vi "save_metadata.vi"(10 "input cluster":T1, 11 "Pasta Destino":path=path "D:/labview_ieav/acquisition") -> ()   [LabVIEW 2020]
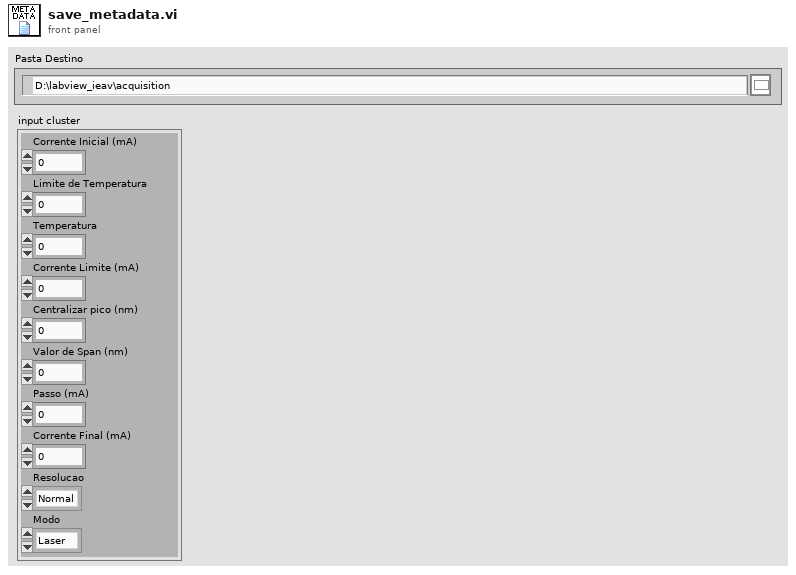
[diagram p1: front panel]
types:
  T1 = cluster{"Corrente Inicial (mA)":dbl, "Limite de Temperatura":dbl, "Temperatura":dbl, "Corrente Limite (mA)":i32, "Centralizar pico (nm)":dbl, "Valor de Span (nm)":dbl, "Passo (mA)":dbl, "Corrente Final (mA)":dbl, "Resolucao":enum16{"Normal", "High"}, "Modo":enum16{"Laser", "Led"}}
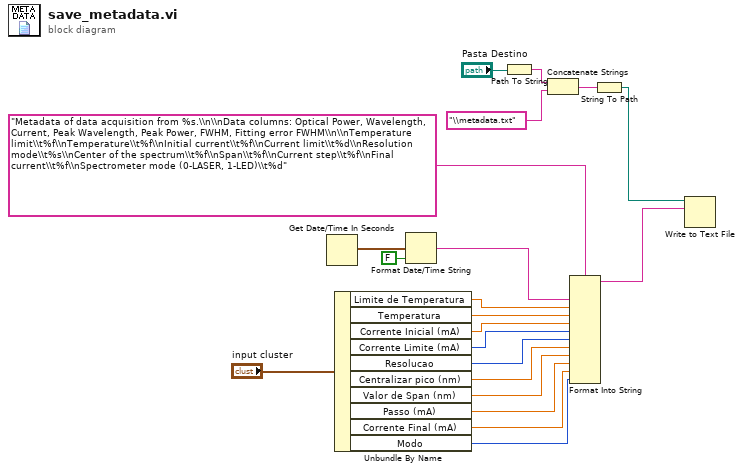
[diagram p0: block diagram]
diagram:
  n1 = Get Date/Time In Seconds() -> (seconds since 1Jan1904=w20:timestamp)
  n2 = Unbundle By Name("input cluster") -> ("Limite de Temperatura"=w18:dbl, "Temperatura"=w17:dbl, "Corrente Inicial (mA)"=w16:dbl, "Corrente Limite (mA)"=w15:i32, "Resolucao"=w14:enum16{"Normal", "High"}, "Centralizar pico (nm)"=w13:dbl, "Valor de Span (nm)"=w12:dbl, "Passo (mA)"=w11:dbl, "Corrente Final (mA)"=w10:dbl, "Modo"=w2:enum16{"Laser", "Led"})
  n3 = Format Date/Time String(seconds (now)=w20, UTC format=FALSE) -> (date/time string=w19:string)  [unwired: 1 in]
  n4 = Path To String(path="Pasta Destino") -> (string=w7:string)
  n5 = Concatenate Strings(w7, "\\metadata.txt") -> (w5:string)
  n6 = Format Into String(format string="Metadata of data acquisition from %s.\\n\\nData columns: Optical Power, Wavelength, Current, Peak Wavelength, Peak Power, FWHM, Fitting error FWHM\\n\\nTemperature limit\\t%f\\nTemperature\\t%f\\nInitial current\\t%f\\nCurrent limit\\t%d\\nResolution mode\\t%s\\nCenter of the spectrum\\t%f\\nSpan\\t%f\\nCurrent step\\t%f\\nFinal current\\t%f\\nSpectrometer mode (0-LASER, 1-LED)\\t%d", w19, w18, w17, w16, w15, w14, w13, w12, w11, w10, w2) -> (resulting string=w21:string)  [unwired: 2 in, 1 out]
  n7 = String To Path(string=w5) -> (path=w4:path)
  n8 = Write to Text File(file (use dialog)=w4, text=w21) -> ()  [unwired: 2 in, 3 out]
